vi "progra ejercicio tania.vi"() -> ()   [LabVIEW 2013]
panel:
  in  "Freno":bool
  in  "Acelerador":bool
  in  "On/Off Auto":bool
  out "Velocidad":dbl(knob) scale=0.0..220.0
  # "Generar la velocidad del auto entre 1-120, luego debemos de\npresionar el acelerador para aumentar la velocidad en 10 y \nal presionar el brake la velocidad bajo 5."
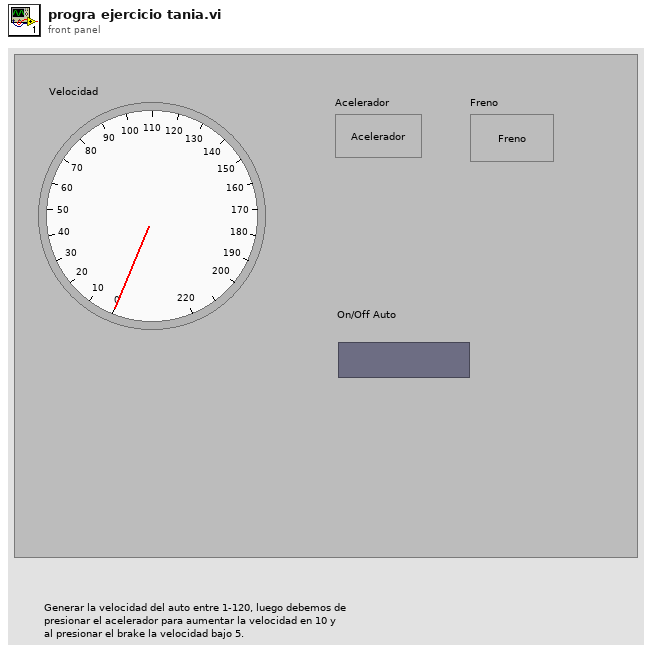
[diagram p1: front panel]
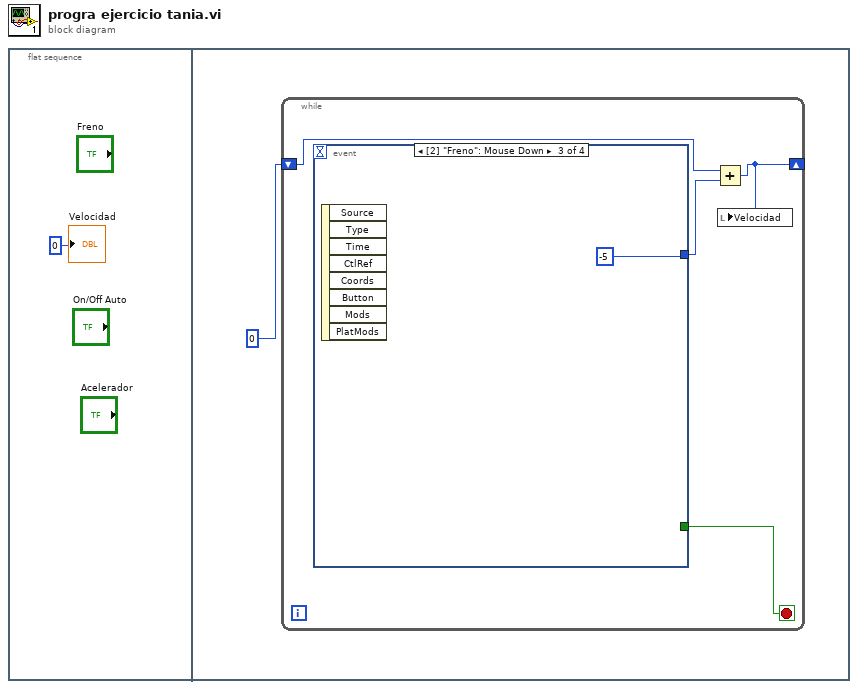
[diagram p0: block diagram]
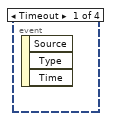
[diagram p2: hidden frame]
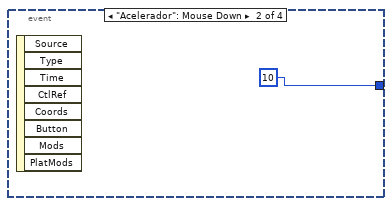
[diagram p3: hidden frame]
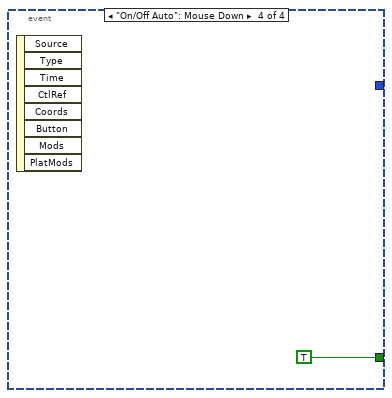
[diagram p4: hidden frame]
diagram:
  n1 = flat-sequence {
    frame #0 {
      "Velocidad" <- 0
    }
    frame #1 {
      n2 = while {
        shift-right: [w4] -> _
        shift-left: 0 -> [w6]
        stop <- w3 stop-if-true
        n3 = event shown="[2] \"Freno\": Mouse Down" {
          selector: _ -> [_ _ _ _]
          dyn-events: _ -> [_ _ _ _]
          timeout: _ -> [_ _ _ _]
          tunnel: [_ 10 -5 _] -> w5
          tunnel: [_ _ _ TRUE] -> w3
          event Timeout {
            n4 = event-data() -> ()  [unwired: 1 in, 3 out]
          }
          event "Acelerador": Mouse Down {
            n5 = event-data() -> ()  [unwired: 1 in, 8 out]
          }
          event "Freno": Mouse Down {
            n6 = event-data() -> ()  [unwired: 1 in, 8 out]
          }
          event "On/Off Auto": Mouse Down {
            n7 = event-data() -> ()  [unwired: 1 in, 8 out]
          }
        }
        n8 = Add(x=w6, y=w5) -> (x+y=w4:i32)
        n9 = local write "Velocidad"(w4) -> ()
      }
    }
  }
